vi "Transfer file to roboRIO.vi"(8 "error in (no error)":errorcluster, 10 "roboRIO Connection Information in":T1, 11 "Configuration File Path":path) -> (0 "error out":errorcluster, 2 "roboRIO Connection Information out":T1, 3 "Status":string)   [LabVIEW 2018, in "Personalities Tool.lvlib"]
doc: "This VI opens a system configuration request to query any roboRIO connected to the computer and sends the file to the first one that it finds."
uses:
  Personalities Tool.lvlib
  Controls/roboRIO Connection Information.ctl
  Controls/Personality Type.ctl
  <vilib>/nisyscfg/Close (System).vi
  <vilib>/Utility/config.llb/Write Key (String).vi
  <vilib>/Utility/config.llb/Write Key (Double).vi
  <vilib>/FTP/NI_FTP.lvlib
  <vilib>/Utility/config.llb/NI_LVConfig.lvlib
  <vilib>/nisyscfg/nisyscfg.lvlib
  <resource>/objmgr/nisysapi.rc
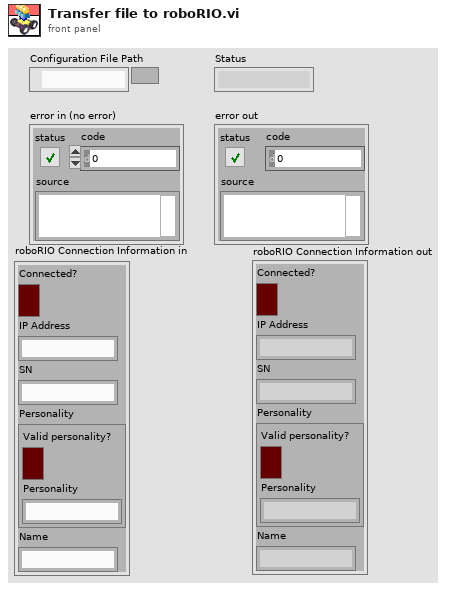
[diagram p1: front panel]
types:
  T1 = typedef "Personalities Tool.lvlib/roboRIO Connection Information.ctl" = cluster{"Connected?":bool, "IP Address":string, "SN":string, "Personality":T2, "Name":string}
  T2 = typedef "Personalities Tool.lvlib/Personality Type.ctl" = cluster{"Valid personality?":bool, "Personality":string}
  T3 = typedef "NI_LVConfig.lvlib/Config Data RefNum.ctl" = refnum<k1>
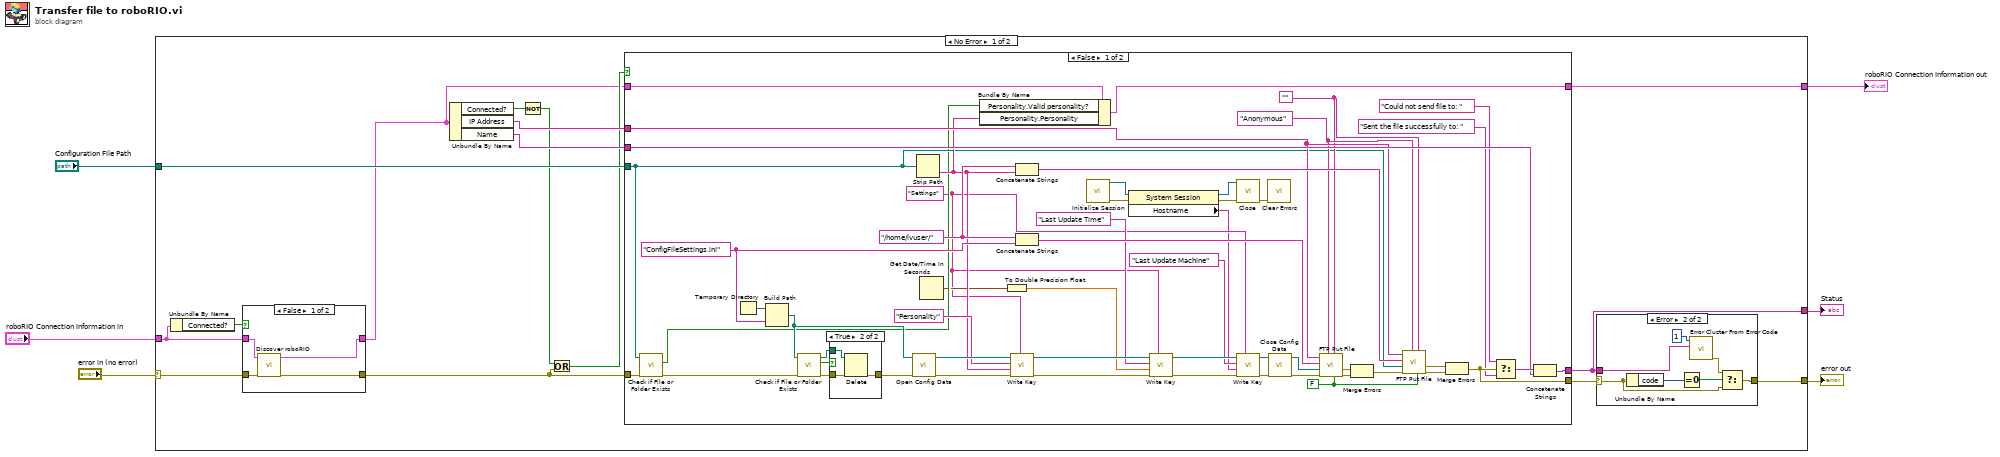
[diagram p0: block diagram]
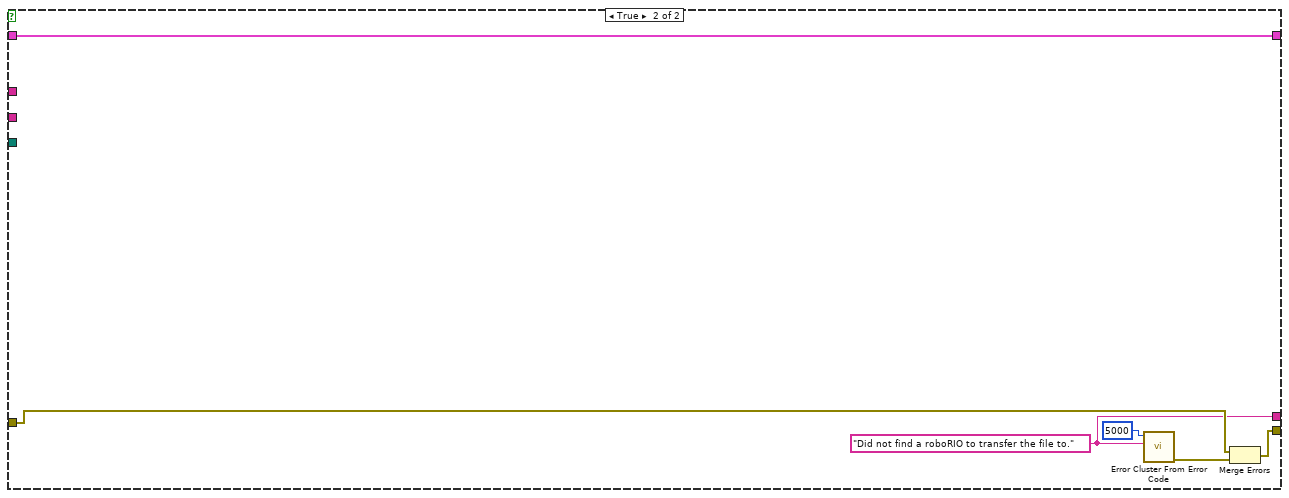
[diagram p5: hidden frame]
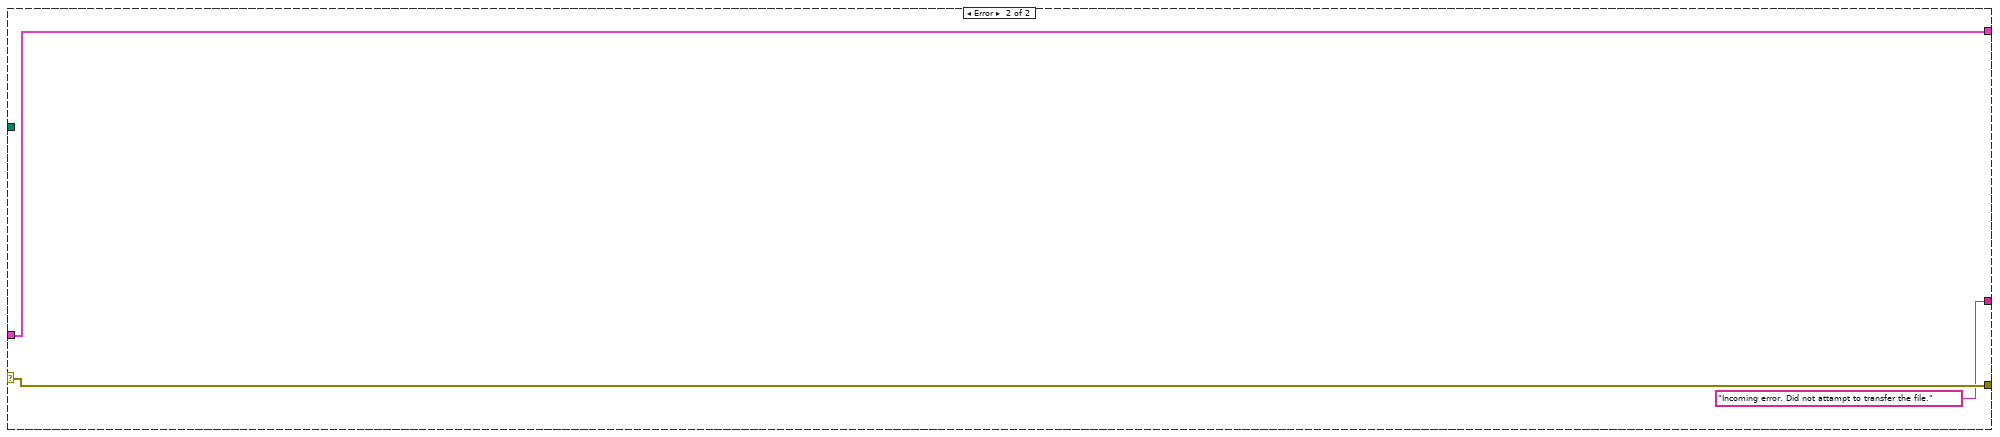
[diagram p6: hidden frame]
diagram:
  n1 = case shown="No Error" "error in (no error)" {
    selector: "error in (no error)" -> [w20 w102]
    tunnel: [w7 "Incoming error. Did not attampt to transfer the file."] -> w6
    tunnel: [w8 w102] -> w5
    tunnel: "Configuration File Path" -> [w21 _]
    tunnel: "roboRIO Connection Information in" -> [w17 w100]
    tunnel: [w10 w100] -> w1
    frame No Error {
      n2 = Unbundle By Name(w17) -> ("Connected?"=w16:bool)
      n3 = case shown="False" w16 {
        tunnel: w20 -> [w33 w35]
        tunnel: [w32 w35] -> w12
        tunnel: w17 -> [w31 w34]
        tunnel: [w30 w34] -> w11
        frame False {
          n4 = call "Discover roboRIO.vi"("error in (no error)"=w33, "roboRIO Connection Information in"=w31) -> ("error out"=w32:errorcluster, "roboRIO Connection Information out"=w30:T1)  [unwired: 8 in]
        }
        frame True {
        }
      }
      n5 = Unbundle By Name(w11) -> ("Connected?"=w14:bool, "IP Address"=w19:string, "Name"=w18:string)
      n6 = Not(x=w14) -> (.not. x?=w13:bool)
      n7 = Or(x=w13, y=w12) -> (x .or. y?=w15:bool)
      n8 = case shown="False" w15 {
        tunnel: w21 -> [w56 _]
        tunnel: [w88 w98] -> w9
        tunnel: w18 -> [w85 _]
        tunnel: w19 -> [w72 _]
        tunnel: [w82 w95] -> w7
        tunnel: w12 -> [w54 w99]
        tunnel: [w58 w94] -> w10
        tunnel: w11 -> [w59 w94]
        frame False {
          w36 = FALSE ("active (T)")
          w44 = "Settings" ("section")
          w61 = "ConfigFileSettings.ini" ("remote path")
          w70 = "" ("password")
          w71 = "Anonymous" ("user")
          w62 = "/home/lvuser/" ("remote path")
          n9 = call <vilib>:"Check if File or Folder Exists.vi"("error in (no error)"=w54, "path"=w56) -> ("error out"=w53:errorcluster, "file or folder exists?"=w55:bool)  [unwired: 7 in, 1 out]
          n10 = Temporary Directory() -> (w68:path)
          n11 = Build Path(base path=w68, name or relative path=w61) -> (appended path=w67:path)
          n12 = call <vilib>:"Check if File or Folder Exists.vi"("error in (no error)"=w53, "path"=w67) -> ("error out"=w65:errorcluster, "file or folder exists?"=w64:bool, "dup path"=w66:path)  [unwired: 7 in]
          n13 = case shown="True" w64 {
            tunnel: w66 -> [_ w93]
            tunnel: w65 -> [w90 w92]
            tunnel: [w90 w91] -> w63
            frame False {
            }
            frame True {
              n14 = Delete(path (use dialog)=w93, error in=w92) -> (error out=w91:errorcluster)  [unwired: 3 in, 2 out]
            }
          }
          n15 = call <vilib>:"Open Config Data.vi"("error in (no error)"=w63, "configuration file path"=w67) -> ("error out"=w79:errorcluster, "refnum"=w80:T3)  [unwired: 7 in, 1 out]
          n16 = Strip Path(path=w56) -> (name=w57:string)  [unwired: 1 out]
          n17 = Get Date/Time In Seconds() -> (seconds since 1Jan1904=w49:timestamp)
          n18 = Bundle By Name(cluster=w59, "Personality.Valid personality?"=w55, "Personality.Personality"=w57) -> (w58:T1)
          n19 = To Double Precision Float(number=w49) -> (double precision float=w48:dbl)
          n20 = call-poly <vilib>:"Write Key.vi"("section"=w44, "error in (no error)"=w79, "value"=w57, "key"="Personality", "refnum"=w80) -> ("error out"=w78:errorcluster, "refnum out"=w51:T3)  [unwired: 4 in, 1 out]
          n21 = Concatenate Strings(w62, w57) -> (w81:string)
          n22 = Concatenate Strings(w62, w61) -> (w60:string)
          n23 = call <vilib>:"Initialize Session.vi"() -> ("error out"=w41:errorcluster, "Session out"=w42:refnum<k21>)  [unwired: 10 in]
          n24 = property class="System Session"(reference=w42, error in=w41) -> (reference out=w40:refnum<k21>, error out=w39:errorcluster, "Hostname"=w38:string)
          n25 = call-poly <vilib>:"Write Key.vi"("section"=w44, "error in (no error)"=w78, "value"=w48, "key"="Last Update Time", "refnum"=w51) -> ("error out"=w52:errorcluster, "refnum out"=w46:T3)  [unwired: 4 in, 1 out]
          n26 = call-poly <vilib>:"Close.vi"("error in (no error)"=w39, "Session in"=w40) -> ("error out"=w37:errorcluster)  [unwired: 9 in]
          n27 = call-poly <vilib>:"Write Key.vi"("section"=w44, "error in (no error)"=w52, "value"=w38, "key"="Last Update Machine", "refnum"=w46) -> ("error out"=w47:errorcluster, "refnum out"=w45:T3)  [unwired: 4 in, 1 out]
          n28 = call <vilib>:"Clear Errors.vi"("error in (no error)"=w37) -> ()  [unwired: 5 in, 2 out]
          n29 = call <vilib>:"Close Config Data.vi"("error in (no error)"=w47, "refnum"=w45) -> ("error out"=w74:errorcluster, "file path"=w73:path)  [unwired: 8 in]
          n30 = call <vilib>:"FTP Put File.vi"("active (T)"=w36, "password"=w70, "user"=w71, "error in (no error)"=w74, "local path"=w73, "remote path"=w60, "host"=w72) -> ("error out"=w75:errorcluster, "file error"=w76:errorcluster)  [unwired: 3 in]
          n31 = Merge Errors(w76, w75) -> (w69:errorcluster)
          n32 = call <vilib>:"FTP Put File.vi"("active (T)"=w36, "password"=w70, "user"=w71, "error in (no error)"=w69, "local path"=w56, "remote path"=w81, "host"=w72) -> ("error out"=w87:errorcluster, "file error"=w86:errorcluster)  [unwired: 3 in]
          n33 = Merge Errors(w86, w87) -> (w88:errorcluster)
          n34 = Select(t="Could not send file to: " ("user"), s=w88, f="Sent the file successfully to: " ("user")) -> (s? t:f=w89:string)
          n35 = Concatenate Strings(w89, w85) -> (w82:string)
        }
        frame True {
          w95 = "Did not find a roboRIO to transfer the file to." ("error message (\"\")")
          n36 = call <vilib>:"Error Cluster From Error Code.vi"("error message (\"\")"=w95, "error code (0)"=5000) -> ("error out"=w97:errorcluster)  [unwired: 7 in]
          n37 = Merge Errors(w99, w97) -> (w98:errorcluster)
        }
      }
      n38 = case shown="Error" w9 {
        selector: w9 -> [w22 w26]
        tunnel: [w22 w27] -> w8
        tunnel: w7 -> [_ w23]
        frame No Error {
        }
        frame Error {
          n39 = Unbundle By Name(w26) -> ("code"=w29:i32)
          n40 = Equal To 0?(x=w29) -> (x = 0?=w28:bool)
          n41 = call <vilib>:"Error Cluster From Error Code.vi"("error message (\"\")"=w23, "error code (0)"=1) -> ("error out"=w25:errorcluster)  [unwired: 7 in]
          n42 = Select(t=w25, s=w28, f=w26) -> (s? t:f=w27:errorcluster)
        }
      }
    }
    frame Error {
    }
  }
  "Status" <- w6
  "error out" <- w5
  "roboRIO Connection Information out" <- w1
